vi "Toggle Boolean Button with the Spacebar LV2012 NI Verified.vi"() -> ()   [LabVIEW 2012]
panel:
  in  "stop":bool
  in  "Boolean":bool
  in  "String":string
  # "Overview: This VI toggles the Boolean button when the space bar pressed, unless the user is entering text into the String Control\nRequirements: LabVIEW 2012 (or compatible)\nInstructions:\n1. Run the VI \n2. Press the spacebar, and notice the Boolean button toggles\n3. Enter a string to the string control. Then press the spacebar, and notice that the boolean button isn't toggling"
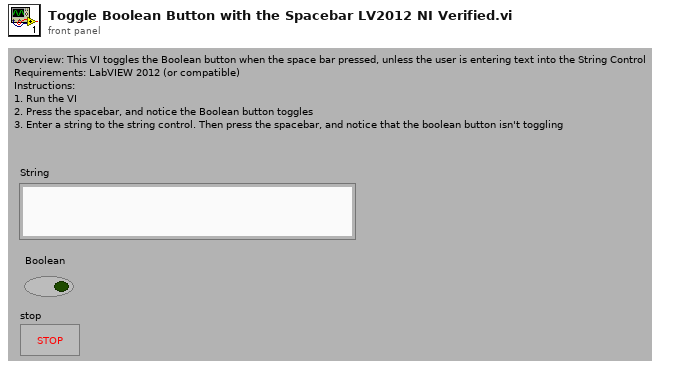
[diagram p1: front panel]
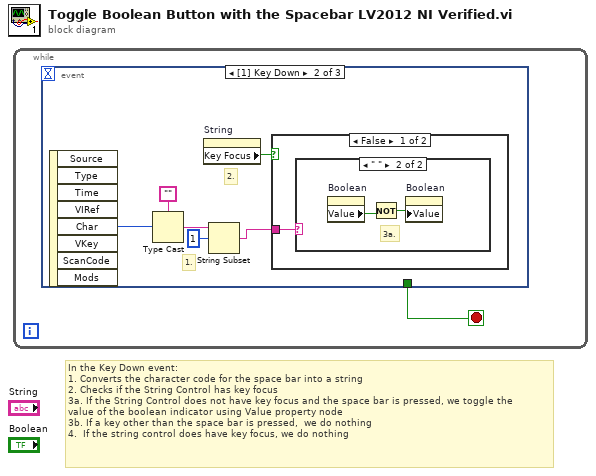
[diagram p0: block diagram]
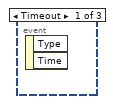
[diagram p2: hidden frame]
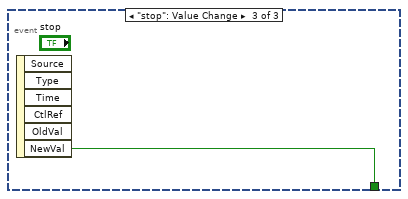
[diagram p5: hidden frame]
diagram:
  # "In the Key Down event:\n1. Converts the character code for the space bar into a string\n2. Checks if the String Control has key focus\n3a. If the String Control does not have key focus and the space bar is pressed, we toggle the     value of the boolean indicator using Value property node  \n3b. If a key other than the space bar is pressed,  we do nothing\n4.  If the string control does have key focus, we do nothing"
  n1 = while {
    stop <- w1 stop-if-true
    n2 = event shown="[1] Key Down" {
      selector: _ -> [_ _ _]
      dyn-events: _ -> [_ _ _]
      timeout: _ -> [_ _ _]
      tunnel: [_ _ w11] -> w1
      event Timeout {
        n3 = event-data() -> ()  [unwired: 1 in, 2 out]
      }
      event Key Down {
        # "2."
        # "1."
        n4 = event-data() -> ("Char"=w7:i16)  [unwired: 1 in, 7 out]
        n5 = Type Cast(type="", x=w7) -> (*(type *) &x=w5:string)
        n6 = property on="String" class="Str"() -> ("Key Focus"=w2:bool)  [unwired: 2 in, 2 out]
        n7 = String Subset(string=w5, offset (0)=1) -> (substring=w3:string)  [unwired: 1 in]
        n8 = case shown="False" w2 {
          tunnel: w3 -> [w8 _]
          frame False {
            n9 = case shown="\" \"" w8 {
              frame "False", Default {
                # "3b."
              }
              frame " " {
                # "3a."
                n10 = property on="Boolean" class="Bool (strict)"() -> ("Value"=w10:bool)  [unwired: 2 in, 2 out]
                n11 = Not(x=w10) -> (.not. x?=w9:bool)
                n12 = property on="Boolean" class="Bool (strict)"("Value"=w9) -> ()  [unwired: 2 in, 2 out]
              }
            }
          }
          frame True {
            # "4."
          }
        }
      }
      event "stop": Value Change {
        n13 = event-data() -> ("NewVal"=w11:bool)  [unwired: 1 in, 5 out]
      }
    }
  }
